vi "MaxCorrelation.vi"(10 "Index in":u16, 11 "Cross Correlation":fxp<+/-,24,8>) -> (1 "Index out":u16, 2 "Numeric":fxp<+/-,33,17>, 3 "Boolean":bool)   [LabVIEW 2015]
uses:
  <vilib>/rvi/DataTransferAndStorage/Container/Common/niFpgaContainerGetUniqueNameForEmu.vi
  <vilib>/rvi/DataTransferAndStorage/Container/Common/niFpgaContainerSetEmuInfo.vi
  <vilib>/rvi/eio/common/nirviEmuReportErrorAndStop.vi
  <vilib>/rvi/DataTransferAndStorage/Container/Common/niFpgaContainerExecOnDevCompGetState.vi
  <vilib>/rvi/Emulation/niFpgaEmulationIsFPGAContextNoSignature.vi
  <vilib>/rvi/Emulation/niFpgaProcessEmulError.vi
  <vilib>/rvi/Emulation/niFpgaSctlEmulationGetInTimedLoop.vi
  <vilib>/rvi/errors/nirviReportUnexpectedCaseInternalError (U32).vi
  <vilib>/rvi/Memory/Memory_Emulation/niFpgaMemoryEmulationCacheClearOnFirstRun.vi
  <vilib>/rvi/Memory/Memory_Emulation/nirvimemoryEmulationManagerCache_MakeExclusive.vi
  <vilib>/rvi/Memory/Memory_Emulation/niFpgaMemoryEmulationValidateCache.vi
  <vilib>/rvi/Memory/Memory_Emulation/nirvimemoryEmulationManagerCache_InsertValue.vi
  <vilib>/Utility/error.llb/Clear Errors.vi
  <vilib>/rvi/Memory/Memory_Emulation/nirvimemoryEmulationManagerCache_ReleaseExclusive.vi
  <vilib>/rvi/Memory/Memory_Emulation/nirvimemoryEmulationManagerCache_GetValue.vi
  <vilib>/rvi/Memory/Memory_Emulation/nirvimemoryEmulationManagerCache_SetValue.vi
  <vilib>/rvi/Emulation/niFpgaSctlEmulationResourceMgr.vi
  <vilib>/rvi/LocalResourceManager/LocalResourceManager.xnode
  <vilib>/rvi/DataTransferAndStorage/Container/XNode/niFpgaContainer.xnode
  <vilib>/rvi/Memory/Memory_Emulation/niFpgaMemoryEmulationRefIn.vi
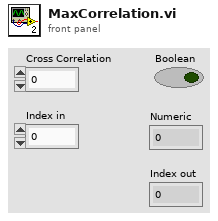
[diagram p1: front panel]
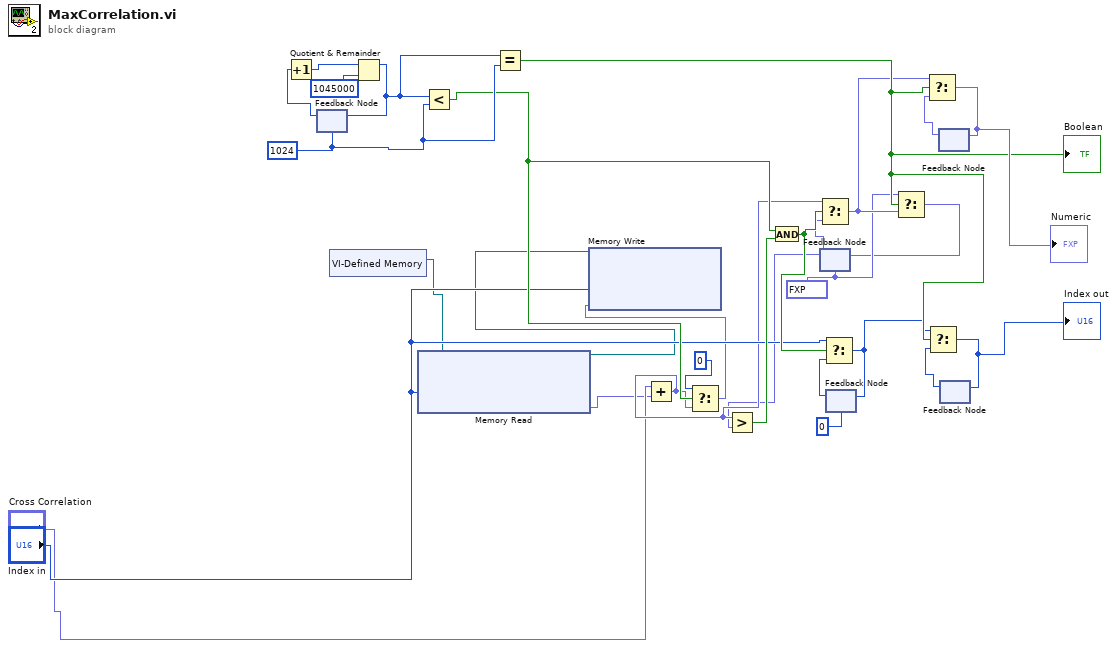
[diagram p0: block diagram]
diagram:
  w16 = fxp<+/-,32,16> -32768.0
  w28 = u64 1024
  n1 = feedback #1(w28) -> (w5:u64)
  n2 = Increment(x=w5) -> (x+1=w6:u64)
  n3 = xnode "VI-Defined Memory"() -> ("Memory Out"=w1:refnum<k21>)
  n4 = Quotient & Remainder(x=w6, y=u64 1045000) -> (x-y*floor(x/y)=w17:u64)  [unwired: 1 out]
  n5 = feedback-in #1(w17) -> ()
  n6 = xnode ("Memory Read")("Address"="Index in", "Memory In"=w1) -> ("Data"=w3:fxp<+/-,32,16>, "Memory Out"=w2:refnum<k21>)
  n7 = Less?(x=w17, y=w28) -> (x < y?=w19:bool)
  n8 = Equal?(x=w17, y=w28) -> (x = y?=w25:bool)
  "Boolean" <- w25
  n9 = Add(x="Cross Correlation", y=w3) -> (x+y=w13:fxp<+/-,33,17>)
  n10 = Select(t=i16 0, s=w19, f=w13) -> (s? t:f=w8:fxp<+/-,33,17>)
  n11 = xnode ("Memory Write")("Address"="Index in", "Data"=w8, "Memory In"=w2) -> ()  [unwired: 1 out]
  n12 = feedback #2(w16) -> (w12:fxp<+/-,33,17>)
  n13 = Greater?(x=w13, y=w12) -> (0:w18:bool)
  n14 = And(x=w19, y=w18) -> (x .and. y?=w20:bool)
  n15 = Select(t=w13, s=w20, f=w12) -> (s? t:f=w24:fxp<+/-,33,17>)
  n16 = feedback #3(u16 0) -> (w11:u16)
  n17 = Select(t="Index in", s=w20, f=w11) -> (s? t:f=w23:u16)
  n18 = feedback-in #3(w23) -> ()
  n19 = Select(t=w16, s=w25, f=w24) -> (s? t:f=w15:fxp<+/-,33,17>)
  n20 = feedback-in #2(w15) -> ()
  n21 = feedback #4() -> (w21:fxp<+/-,33,17>)  [unwired: 1 in]
  n22 = Select(t=w24, s=w25, f=w21) -> (s? t:f=w27:fxp<+/-,33,17>)
  "Numeric" <- w27
  n23 = feedback-in #4(w27) -> ()
  n24 = feedback #5() -> (w22:u16)  [unwired: 1 in]
  n25 = Select(t=w23, s=w25, f=w22) -> (s? t:f=w26:u16)
  "Index out" <- w26
  n26 = feedback-in #5(w26) -> ()
